vi "Init File Storage.vi"(8 "error in (no error)":errorcluster, 11 "Session Storage Folder":path) -> (0 "error out":errorcluster, 3 "Session out":refnum<class "Session.lvclass">)   [LabVIEW 2020, in "HTTP Server.lvlib" / "Session.lvclass"]
doc: "Initializes a local folder for storing session data. The specified folder must already exist otherwise an error will be generated when trying to register the session implementation with the server."
uses:
  Session.lvclass
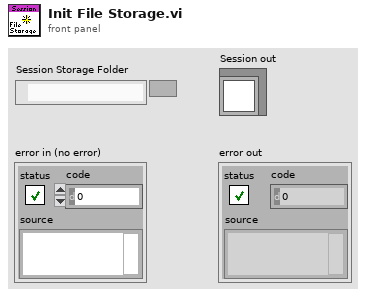
[diagram p1: front panel]
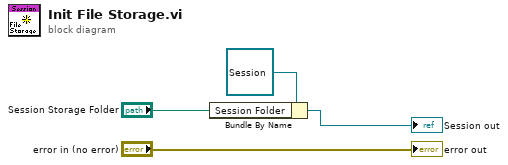
[diagram p0: block diagram]
diagram:
  n1 = Bundle By Name(cluster=refnum<class "Session.lvclass"> refnum ("Session in"), "Session Folder"="Session Storage Folder") -> (→"Session out":refnum<class "Session.lvclass">)
  "error out" <- "error in (no error)"
